vi "getMoveParametersAllAxis.vi"(8 "error":errorcluster, 11 "connection ID":refnum<k5>) -> (0 "error out":errorcluster, 2 "MoveParameters":T1, 3 "connection ID out":refnum<k5>)   [LabVIEW 2016, in "AMC_VIs.lvlib"]
doc: "This function reads the parameters for controling the positioners on all three axes\nThe parameters are ampltidue (V), sawtooth-frequency (Hz), currently on the piezo applied voltage (V)\nControl function\nInputs:\n none\nOutputs: err\n amplitude_ax1_mV\n frequency_ax1_mHz\n appliedVoltage_ax1_mV currently applied \"DC\"-Voltage\n amplitude_ax2_mV\n frequency_ax2_mHz\n appliedVoltage_ax2_mV currently applied \"DC\"-Voltage\n amplitude_ax3_mV\n frequency_ax3_mHz\n appliedVoltage_ax3_mV currently applied \"DC\"-Voltage"
uses:
  AMC_VIs.lvlib
panel:
  out "JSON-response":string="{\"jsonrpc\":\"2.0\",\"method\":\"\",\"params\":[5,1.245,true,\"name\"],\"id\":\"1\"}"
  out "JSON request":string
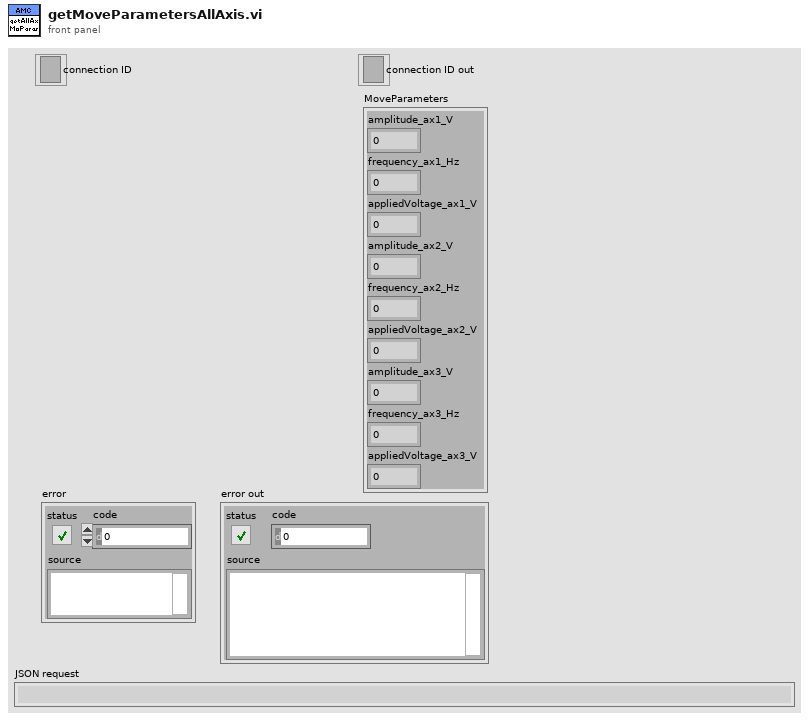
[diagram p1: front panel]
types:
  T1 = cluster{"amplitude_ax1_V":dbl, "frequency_ax1_Hz":dbl, "appliedVoltage_ax1_V":dbl, "amplitude_ax2_V":dbl, "frequency_ax2_Hz":dbl, "appliedVoltage_ax2_V":dbl, "amplitude_ax3_V":dbl, "frequency_ax3_Hz":dbl, "appliedVoltage_ax3_V":dbl}
  T2 = cluster{"jsonrpc":string, "method":string, "params":i32[], "id":string, "api":string}
  T3 = cluster{"jsonrpc":string, "result":i32[], "id":string}
  T4 = enum16{"Standard", "Buffered", "CRLF", "Immediate"}
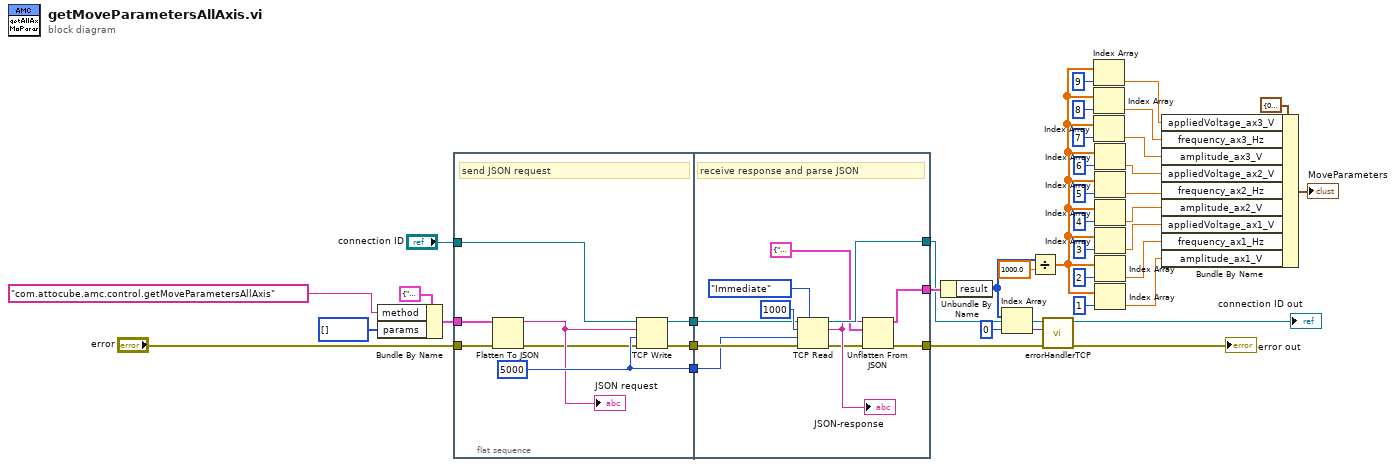
[diagram p0: block diagram]
diagram:
  n1 = Bundle By Name(cluster=T2 {"jsonrpc"="2.0", "method"="com.attocube.amc.res.setRESReadOutFreq", "params"=[0, 2712], "id"="1", "api"="2"} ("InputParams 2"), "method"="com.attocube.amc.control.getMoveParametersAllAxis", "params"=i32[] []) -> (w32:T2)
  n2 = flat-sequence {
    tunnel: "connection ID" -> [w47]
    tunnel: [w45] -> w39
    tunnel: [w46] -> w38
    tunnel: "error" -> [w41]
    tunnel: [w44] -> w37
    tunnel: w32 -> [w43]
    tunnel: [w54] -> w25
    tunnel: w39 -> [w56]
    tunnel: w38 -> [w55]
    tunnel: [w50] -> w28
    tunnel: w37 -> [w53]
    tunnel: [w49] -> w31
    frame #0 {
      w44 = 5000 ("timeout ms (25000)")
      # "send JSON request"
      n3 = Flatten To JSON(anything=w43, error in (no error)=w41) -> (JSON string=w42:string, 11:w40:errorcluster)  [unwired: 1 in]
      "JSON request" <- w42
      n4 = TCP Write(connection ID=w47, data in=w42, error in (no error)=w40, 9:w44) -> (connection ID out=w45:refnum<k5>, error out=w46:errorcluster)  [unwired: 1 out]
    }
    frame #1 {
      # "receive response and parse JSON"
      n5 = TCP Read(connection ID=w56, bytes to read=1000, error in (no error)=w55, 7:T4."Immediate" ("mode (standard)"), 9:w53) -> (connection ID out=w54:refnum<k5>, data out=w52:string, error out=w51:errorcluster)
      "JSON-response" <- w52
      n6 = Unflatten From JSON(JSON string=w52, type and defaults=T3 {"jsonrpc"="2.0", "result"=[0, 2712], "id"="1"} ("InputParams 2"), error in (no error)=w51) -> (value=w49:T3, error out=w50:errorcluster)  [unwired: 4 in]
    }
  }
  n7 = Unbundle By Name(w31) -> ("result"=w2:i32[])
  n8 = Index Array(array=w2, index=0) -> (element=w27:i32)
  n9 = Divide(x=w2, y=1000.0) -> (x/y=w1:dbl[])
  n10 = call "errorHandlerTCP.vi"("error in"=w28, "error number"=w27, "connection ID"=w25) -> ("error out"=→"error out":errorcluster, "connection ID"=→"connection ID out":refnum<k5>)  [unwired: 7 in]
  n11 = Index Array(array=w1, index=9) -> (element=w12:dbl)
  n12 = Index Array(array=w1, index=8) -> (element=w4:dbl)
  n13 = Index Array(array=w1, index=7) -> (element=w5:dbl)
  n14 = Index Array(array=w1, index=6) -> (element=w6:dbl)
  n15 = Index Array(array=w1, index=5) -> (element=w7:dbl)
  n16 = Index Array(array=w1, index=4) -> (element=w8:dbl)
  n17 = Index Array(array=w1, index=3) -> (element=w9:dbl)
  n18 = Index Array(array=w1, index=2) -> (element=w10:dbl)
  n19 = Index Array(array=w1, index=1) -> (element=w11:dbl)
  n20 = Bundle By Name(cluster=T1 {"amplitude_ax1_V"=0.0, "frequency_ax1_Hz"=0.0, "appliedVoltage_ax1_V"=0.0, "amplitude_ax2_V"=0.0, "frequency_ax2_Hz"=0.0, "appliedVoltage_ax2_V"=0.0, "amplitude_ax3_V"=0.0, "frequency_ax3_Hz"=0.0, "appliedVoltage_ax3_V"=0.0}, "appliedVoltage_ax3_V"=w12, "frequency_ax3_Hz"=w4, "amplitude_ax3_V"=w5, "appliedVoltage_ax2_V"=w6, "frequency_ax2_Hz"=w7, "amplitude_ax2_V"=w8, "appliedVoltage_ax1_V"=w9, "frequency_ax1_Hz"=w10, "amplitude_ax1_V"=w11) -> (→"MoveParameters":T1)
